vi "G2CPU Circle Lines.vi"(6 "Auto Release (Enabled)":T2={"Auto Release Amount of Lines (Enabled)"=TRUE, "Auto Release Center X (Enabled)"=TRUE, "Auto Release Center Y (Enabled)"=TRUE, "Auto Release Inner Radius (Enabled)"=TRUE, "Auto Release Outer Radius (Enabled)"=TRUE}, 8 "error in (no error)":errorcluster, 11 "Circles Parameters":T1) -> (0 "error out":errorcluster, 3 "Lines":T3)   [LabVIEW 2020, in "G2CPU Line Profile.lvlib"]
doc: "Create a set of points representing a set of Circles for image processing.\n\nPoints 1 on the output define the starting point of the lines and Points 2 define the stopping point of the lines.\nThe keys put out define the grouping of the lines to each circle."
uses:
  G2CPU Line Profile.lvlib
  <vilib>/Natan Biesmans/G2CPU GPU and CPU HPC Toolkit/G2CPU Libraries/Arrays/1DArray/f32/1D Array f32.lvclass
  C:/Program Files/National Instruments/LabVIEW 2025/vi.lib/Natan Biesmans/G2CPU GPU and CPU HPC Toolkit/G2CPU Libraries/Arrays/Array/Array Prototype.lvclass
  <vilib>/Natan Biesmans/G2CPU GPU and CPU HPC Toolkit/G2CPU Libraries/Arrays/1DArray/u32/1D Array u32.lvclass
  <vilib>/Natan Biesmans/G2CPU GPU and CPU HPC Toolkit/G2CPU Libraries/Arrays/1DArray/s32/1D Array s32.lvclass
  <vilib>/Natan Biesmans/G2CPU GPU and CPU HPC Toolkit/G2CPU Libraries/Arrays/Array/Array Prototype.lvclass/Array Prototype.ctl
  5b6760fa-9266-4741-afe7-4312c65416e9.vi
  3ad29c53-26f3-45f8-97d6-314157a676f7.vi
  14fba4ab-b554-44ef-a6f4-b6fd1a5d0cda.vi
  d3b3dbab-8883-4f98-9cce-319203c44813.vi
  e6c5d5d9-651a-47bf-ad11-961ed0f765a8.vi
  89c6f82f-ffef-4584-9d82-73d0fa6da3da.vi
  6a456209-1d8e-4cf0-9b04-3ffbd32bc9ac.vi
  96931e95-d0f5-44f7-b248-8357b3156dd5.vi
  d7ba55f0-9849-4505-a6fd-be5dcb5421fd.vi
  1cc5007f-c24b-4d5b-aa75-be27a96b3985.vi
  9a111955-ab15-448a-9318-e20ab5826a62.vi
  6db02158-8bc6-4d9a-a007-839d85d2f15d.vi
  ec8ba2e3-79c6-4f50-951d-f45e21c11e8a.vi
  f4669a4f-8dee-47e0-9080-20b8edd3c1cc.vi
  7ced169a-8142-4f3b-944f-65e1b7c596f5.vi
  2317dfd0-6b1c-49a0-9577-73dec4764c65.vi
  <vilib>/Natan Biesmans/G2CPU GPU and CPU HPC Toolkit/G2CPU Libraries/Arrays/Array/G2CPU Get Array Pointer.vi
  5b6760fa-9266-4741-afe7-4312c65416e9.vi/10d88d95-1d79-457d-a71e-58ed0fd5ba1c.vi
  3ad29c53-26f3-45f8-97d6-314157a676f7.vi/266dcd25-0bcc-42fd-b83c-a48544f38d1c.vi
  14fba4ab-b554-44ef-a6f4-b6fd1a5d0cda.vi/6197f869-f6d4-49b3-9b2c-cc979b422c2e.vi
  14fba4ab-b554-44ef-a6f4-b6fd1a5d0cda.vi/a7e86dbb-b4c0-485c-89c5-522e60ee265c.vi
  d3b3dbab-8883-4f98-9cce-319203c44813.vi/6197f869-f6d4-49b3-9b2c-cc979b422c2e.vi
  d3b3dbab-8883-4f98-9cce-319203c44813.vi/a7e86dbb-b4c0-485c-89c5-522e60ee265c.vi
  e6c5d5d9-651a-47bf-ad11-961ed0f765a8.vi/6197f869-f6d4-49b3-9b2c-cc979b422c2e.vi
  e6c5d5d9-651a-47bf-ad11-961ed0f765a8.vi/a7e86dbb-b4c0-485c-89c5-522e60ee265c.vi
  89c6f82f-ffef-4584-9d82-73d0fa6da3da.vi/6197f869-f6d4-49b3-9b2c-cc979b422c2e.vi
  89c6f82f-ffef-4584-9d82-73d0fa6da3da.vi/a7e86dbb-b4c0-485c-89c5-522e60ee265c.vi
  6a456209-1d8e-4cf0-9b04-3ffbd32bc9ac.vi/5793b77b-c002-4ebf-9075-685617c95341.vi
  6a456209-1d8e-4cf0-9b04-3ffbd32bc9ac.vi/2ed3ef86-c00d-4d71-b84c-20267a6dfcf9.vi
  96931e95-d0f5-44f7-b248-8357b3156dd5.vi/5793b77b-c002-4ebf-9075-685617c95341.vi
  96931e95-d0f5-44f7-b248-8357b3156dd5.vi/2ed3ef86-c00d-4d71-b84c-20267a6dfcf9.vi
  d7ba55f0-9849-4505-a6fd-be5dcb5421fd.vi/5793b77b-c002-4ebf-9075-685617c95341.vi
  d7ba55f0-9849-4505-a6fd-be5dcb5421fd.vi/2ed3ef86-c00d-4d71-b84c-20267a6dfcf9.vi
  1cc5007f-c24b-4d5b-aa75-be27a96b3985.vi/5793b77b-c002-4ebf-9075-685617c95341.vi
  1cc5007f-c24b-4d5b-aa75-be27a96b3985.vi/2ed3ef86-c00d-4d71-b84c-20267a6dfcf9.vi
  9a111955-ab15-448a-9318-e20ab5826a62.vi/e9bebd79-1c27-4fc1-b91f-30516104c7f0.vi
  6db02158-8bc6-4d9a-a007-839d85d2f15d.vi/7467a0f1-0650-4e63-b635-b3d2b2ec9a4e.vi
  6db02158-8bc6-4d9a-a007-839d85d2f15d.vi/8ee11bc3-5ef5-497e-97f0-8db2b3aaa149.vi
  6db02158-8bc6-4d9a-a007-839d85d2f15d.vi/c7af9698-5e3c-4e11-95da-3024075b67d2.vi
  ec8ba2e3-79c6-4f50-951d-f45e21c11e8a.vi/a7ec311c-7cd8-4650-9526-d70ff0a769d1.vi
  f4669a4f-8dee-47e0-9080-20b8edd3c1cc.vi/e9bebd79-1c27-4fc1-b91f-30516104c7f0.vi
  7ced169a-8142-4f3b-944f-65e1b7c596f5.vi/7467a0f1-0650-4e63-b635-b3d2b2ec9a4e.vi
  7ced169a-8142-4f3b-944f-65e1b7c596f5.vi/8ee11bc3-5ef5-497e-97f0-8db2b3aaa149.vi
  7ced169a-8142-4f3b-944f-65e1b7c596f5.vi/c7af9698-5e3c-4e11-95da-3024075b67d2.vi
  2317dfd0-6b1c-49a0-9577-73dec4764c65.vi/2e03f477-51b7-4ba0-bb4f-4f838f6557e6.vi
  2317dfd0-6b1c-49a0-9577-73dec4764c65.vi/125d45d4-836b-469d-8a4a-6adb452f866d.vi
  2317dfd0-6b1c-49a0-9577-73dec4764c65.vi/8038e9ed-2e71-4568-91ba-0d873494c5ed.vi
  14fba4ab-b554-44ef-a6f4-b6fd1a5d0cda.vi/6197f869-f6d4-49b3-9b2c-cc979b422c2e.vi/3e802c67-fb96-46a3-ae13-4994a8508b4f.vi
  14fba4ab-b554-44ef-a6f4-b6fd1a5d0cda.vi/6197f869-f6d4-49b3-9b2c-cc979b422c2e.vi/5a50fc67-79e7-4972-80c2-92243cd53dd4.vi
  14fba4ab-b554-44ef-a6f4-b6fd1a5d0cda.vi/a7e86dbb-b4c0-485c-89c5-522e60ee265c.vi/730f6c57-5c0b-4ee9-b61e-75067b25222b.vi
  14fba4ab-b554-44ef-a6f4-b6fd1a5d0cda.vi/a7e86dbb-b4c0-485c-89c5-522e60ee265c.vi/096b8799-7810-404e-baca-ba9279cec4bd.vi
  14fba4ab-b554-44ef-a6f4-b6fd1a5d0cda.vi/a7e86dbb-b4c0-485c-89c5-522e60ee265c.vi/0f1a5a47-bcc5-4796-ac31-8dfcfbc0d7d1.vi
  14fba4ab-b554-44ef-a6f4-b6fd1a5d0cda.vi/a7e86dbb-b4c0-485c-89c5-522e60ee265c.vi/89f12e17-3330-4b72-ad8f-8dd636660732.vi
  d3b3dbab-8883-4f98-9cce-319203c44813.vi/6197f869-f6d4-49b3-9b2c-cc979b422c2e.vi/3e802c67-fb96-46a3-ae13-4994a8508b4f.vi
  d3b3dbab-8883-4f98-9cce-319203c44813.vi/6197f869-f6d4-49b3-9b2c-cc979b422c2e.vi/5a50fc67-79e7-4972-80c2-92243cd53dd4.vi
  d3b3dbab-8883-4f98-9cce-319203c44813.vi/a7e86dbb-b4c0-485c-89c5-522e60ee265c.vi/730f6c57-5c0b-4ee9-b61e-75067b25222b.vi
  d3b3dbab-8883-4f98-9cce-319203c44813.vi/a7e86dbb-b4c0-485c-89c5-522e60ee265c.vi/096b8799-7810-404e-baca-ba9279cec4bd.vi
  d3b3dbab-8883-4f98-9cce-319203c44813.vi/a7e86dbb-b4c0-485c-89c5-522e60ee265c.vi/0f1a5a47-bcc5-4796-ac31-8dfcfbc0d7d1.vi
  d3b3dbab-8883-4f98-9cce-319203c44813.vi/a7e86dbb-b4c0-485c-89c5-522e60ee265c.vi/89f12e17-3330-4b72-ad8f-8dd636660732.vi
  e6c5d5d9-651a-47bf-ad11-961ed0f765a8.vi/6197f869-f6d4-49b3-9b2c-cc979b422c2e.vi/3e802c67-fb96-46a3-ae13-4994a8508b4f.vi
  e6c5d5d9-651a-47bf-ad11-961ed0f765a8.vi/6197f869-f6d4-49b3-9b2c-cc979b422c2e.vi/5a50fc67-79e7-4972-80c2-92243cd53dd4.vi
  e6c5d5d9-651a-47bf-ad11-961ed0f765a8.vi/a7e86dbb-b4c0-485c-89c5-522e60ee265c.vi/730f6c57-5c0b-4ee9-b61e-75067b25222b.vi
  e6c5d5d9-651a-47bf-ad11-961ed0f765a8.vi/a7e86dbb-b4c0-485c-89c5-522e60ee265c.vi/096b8799-7810-404e-baca-ba9279cec4bd.vi
  e6c5d5d9-651a-47bf-ad11-961ed0f765a8.vi/a7e86dbb-b4c0-485c-89c5-522e60ee265c.vi/0f1a5a47-bcc5-4796-ac31-8dfcfbc0d7d1.vi
  e6c5d5d9-651a-47bf-ad11-961ed0f765a8.vi/a7e86dbb-b4c0-485c-89c5-522e60ee265c.vi/89f12e17-3330-4b72-ad8f-8dd636660732.vi
  89c6f82f-ffef-4584-9d82-73d0fa6da3da.vi/6197f869-f6d4-49b3-9b2c-cc979b422c2e.vi/3e802c67-fb96-46a3-ae13-4994a8508b4f.vi
  89c6f82f-ffef-4584-9d82-73d0fa6da3da.vi/6197f869-f6d4-49b3-9b2c-cc979b422c2e.vi/5a50fc67-79e7-4972-80c2-92243cd53dd4.vi
  89c6f82f-ffef-4584-9d82-73d0fa6da3da.vi/a7e86dbb-b4c0-485c-89c5-522e60ee265c.vi/730f6c57-5c0b-4ee9-b61e-75067b25222b.vi
  89c6f82f-ffef-4584-9d82-73d0fa6da3da.vi/a7e86dbb-b4c0-485c-89c5-522e60ee265c.vi/096b8799-7810-404e-baca-ba9279cec4bd.vi
  89c6f82f-ffef-4584-9d82-73d0fa6da3da.vi/a7e86dbb-b4c0-485c-89c5-522e60ee265c.vi/0f1a5a47-bcc5-4796-ac31-8dfcfbc0d7d1.vi
  89c6f82f-ffef-4584-9d82-73d0fa6da3da.vi/a7e86dbb-b4c0-485c-89c5-522e60ee265c.vi/89f12e17-3330-4b72-ad8f-8dd636660732.vi
  6a456209-1d8e-4cf0-9b04-3ffbd32bc9ac.vi/5793b77b-c002-4ebf-9075-685617c95341.vi/3e802c67-fb96-46a3-ae13-4994a8508b4f.vi
  6a456209-1d8e-4cf0-9b04-3ffbd32bc9ac.vi/5793b77b-c002-4ebf-9075-685617c95341.vi/5a50fc67-79e7-4972-80c2-92243cd53dd4.vi
  6a456209-1d8e-4cf0-9b04-3ffbd32bc9ac.vi/2ed3ef86-c00d-4d71-b84c-20267a6dfcf9.vi/730f6c57-5c0b-4ee9-b61e-75067b25222b.vi
  6a456209-1d8e-4cf0-9b04-3ffbd32bc9ac.vi/2ed3ef86-c00d-4d71-b84c-20267a6dfcf9.vi/096b8799-7810-404e-baca-ba9279cec4bd.vi
  6a456209-1d8e-4cf0-9b04-3ffbd32bc9ac.vi/2ed3ef86-c00d-4d71-b84c-20267a6dfcf9.vi/0f1a5a47-bcc5-4796-ac31-8dfcfbc0d7d1.vi
  6a456209-1d8e-4cf0-9b04-3ffbd32bc9ac.vi/2ed3ef86-c00d-4d71-b84c-20267a6dfcf9.vi/89f12e17-3330-4b72-ad8f-8dd636660732.vi
  96931e95-d0f5-44f7-b248-8357b3156dd5.vi/5793b77b-c002-4ebf-9075-685617c95341.vi/3e802c67-fb96-46a3-ae13-4994a8508b4f.vi
  96931e95-d0f5-44f7-b248-8357b3156dd5.vi/5793b77b-c002-4ebf-9075-685617c95341.vi/5a50fc67-79e7-4972-80c2-92243cd53dd4.vi
  96931e95-d0f5-44f7-b248-8357b3156dd5.vi/2ed3ef86-c00d-4d71-b84c-20267a6dfcf9.vi/730f6c57-5c0b-4ee9-b61e-75067b25222b.vi
  96931e95-d0f5-44f7-b248-8357b3156dd5.vi/2ed3ef86-c00d-4d71-b84c-20267a6dfcf9.vi/096b8799-7810-404e-baca-ba9279cec4bd.vi
  96931e95-d0f5-44f7-b248-8357b3156dd5.vi/2ed3ef86-c00d-4d71-b84c-20267a6dfcf9.vi/0f1a5a47-bcc5-4796-ac31-8dfcfbc0d7d1.vi
  96931e95-d0f5-44f7-b248-8357b3156dd5.vi/2ed3ef86-c00d-4d71-b84c-20267a6dfcf9.vi/89f12e17-3330-4b72-ad8f-8dd636660732.vi
  d7ba55f0-9849-4505-a6fd-be5dcb5421fd.vi/5793b77b-c002-4ebf-9075-685617c95341.vi/3e802c67-fb96-46a3-ae13-4994a8508b4f.vi
  d7ba55f0-9849-4505-a6fd-be5dcb5421fd.vi/5793b77b-c002-4ebf-9075-685617c95341.vi/5a50fc67-79e7-4972-80c2-92243cd53dd4.vi
  d7ba55f0-9849-4505-a6fd-be5dcb5421fd.vi/2ed3ef86-c00d-4d71-b84c-20267a6dfcf9.vi/730f6c57-5c0b-4ee9-b61e-75067b25222b.vi
  d7ba55f0-9849-4505-a6fd-be5dcb5421fd.vi/2ed3ef86-c00d-4d71-b84c-20267a6dfcf9.vi/096b8799-7810-404e-baca-ba9279cec4bd.vi
  d7ba55f0-9849-4505-a6fd-be5dcb5421fd.vi/2ed3ef86-c00d-4d71-b84c-20267a6dfcf9.vi/0f1a5a47-bcc5-4796-ac31-8dfcfbc0d7d1.vi
  d7ba55f0-9849-4505-a6fd-be5dcb5421fd.vi/2ed3ef86-c00d-4d71-b84c-20267a6dfcf9.vi/89f12e17-3330-4b72-ad8f-8dd636660732.vi
  1cc5007f-c24b-4d5b-aa75-be27a96b3985.vi/5793b77b-c002-4ebf-9075-685617c95341.vi/3e802c67-fb96-46a3-ae13-4994a8508b4f.vi
  1cc5007f-c24b-4d5b-aa75-be27a96b3985.vi/5793b77b-c002-4ebf-9075-685617c95341.vi/5a50fc67-79e7-4972-80c2-92243cd53dd4.vi
  1cc5007f-c24b-4d5b-aa75-be27a96b3985.vi/2ed3ef86-c00d-4d71-b84c-20267a6dfcf9.vi/730f6c57-5c0b-4ee9-b61e-75067b25222b.vi
  1cc5007f-c24b-4d5b-aa75-be27a96b3985.vi/2ed3ef86-c00d-4d71-b84c-20267a6dfcf9.vi/096b8799-7810-404e-baca-ba9279cec4bd.vi
  1cc5007f-c24b-4d5b-aa75-be27a96b3985.vi/2ed3ef86-c00d-4d71-b84c-20267a6dfcf9.vi/0f1a5a47-bcc5-4796-ac31-8dfcfbc0d7d1.vi
  1cc5007f-c24b-4d5b-aa75-be27a96b3985.vi/2ed3ef86-c00d-4d71-b84c-20267a6dfcf9.vi/89f12e17-3330-4b72-ad8f-8dd636660732.vi
  2317dfd0-6b1c-49a0-9577-73dec4764c65.vi/2e03f477-51b7-4ba0-bb4f-4f838f6557e6.vi/d8e2d9cc-c923-495e-b121-b6b84788c73f.vi
  2317dfd0-6b1c-49a0-9577-73dec4764c65.vi/2e03f477-51b7-4ba0-bb4f-4f838f6557e6.vi/345e91f0-9a5e-4de4-af9c-133346717e4a.vi
  <vilib>/Natan Biesmans/G2CPU GPU and CPU HPC Toolkit/G2CPU Libraries/Arrays/2DArray/f32/2D Array f32.lvclass
  <vilib>/Natan Biesmans/G2CPU GPU and CPU HPC Toolkit/G2CPU Libraries/Arrays/2DArray/binary/2D Array binary.lvclass
  <vilib>/Natan Biesmans/G2CPU GPU and CPU HPC Toolkit/G2CPU Libraries/Arrays/1DArray/binary/1D Array binary.lvclass
  <vilib>/Natan Biesmans/G2CPU GPU and CPU HPC Toolkit/G2CPU Libraries/Arrays/2DArray/u32/2D Array u32.lvclass
  <vilib>/Natan Biesmans/G2CPU GPU and CPU HPC Toolkit/ArrayFire Driver/VIs/cos.vi
  <vilib>/Natan Biesmans/G2CPU GPU and CPU HPC Toolkit/G2CPU Libraries/Arrays/Array/G2CPU Set Array Pointer.vi
  <vilib>/Natan Biesmans/G2CPU GPU and CPU HPC Toolkit/ArrayFire Driver/VIs/sin.vi
  <vilib>/Natan Biesmans/G2CPU GPU and CPU HPC Toolkit/G2CPU Libraries/Arrays/SubVI/is 2D.vi
  <vilib>/Natan Biesmans/G2CPU GPU and CPU HPC Toolkit/ArrayFire Driver/VIs/mul.vi
  <vilib>/Natan Biesmans/G2CPU GPU and CPU HPC Toolkit/ArrayFire Driver/VIs/add.vi
  <vilib>/Natan Biesmans/G2CPU GPU and CPU HPC Toolkit/ArrayFire Driver/VIs/transpose.vi
  <vilib>/Natan Biesmans/G2CPU GPU and CPU HPC Toolkit/ArrayFire Driver/VIs/flat.vi
  <vilib>/Natan Biesmans/G2CPU GPU and CPU HPC Toolkit/ArrayFire Driver/VIs/where.vi
  <vilib>/Natan Biesmans/G2CPU GPU and CPU HPC Toolkit/ArrayFire Driver/VIs/cast.vi
  <vilib>/Natan Biesmans/G2CPU GPU and CPU HPC Toolkit/ArrayFire Driver/VIs/lookup.vi
  <vilib>/Natan Biesmans/G2CPU GPU and CPU HPC Toolkit/G2CPU Libraries/Arrays/Array/Array Prototype.lvclass
  <vilib>/Natan Biesmans/G2CPU GPU and CPU HPC Toolkit/G2CPU Libraries/Arrays/DataTypes/f32/f32.lvclass
  <vilib>/Natan Biesmans/G2CPU GPU and CPU HPC Toolkit/G2CPU Libraries/Arrays/2DArray/2D Array Prototype.lvclass
  <vilib>/Natan Biesmans/G2CPU GPU and CPU HPC Toolkit/G2CPU Libraries/Arrays/1DArray/1D Array Prototype.lvclass
  <vilib>/Natan Biesmans/G2CPU GPU and CPU HPC Toolkit/G2CPU Libraries/Arrays/DataTypes/Boolean/Boolean.lvclass
  <vilib>/Natan Biesmans/G2CPU GPU and CPU HPC Toolkit/G2CPU Libraries/Arrays/DataTypes/U32/U32.lvclass
  <vilib>/Natan Biesmans/G2CPU GPU and CPU HPC Toolkit/G2CPU Libraries/Arrays/DataTypes/I32/s32.lvclass
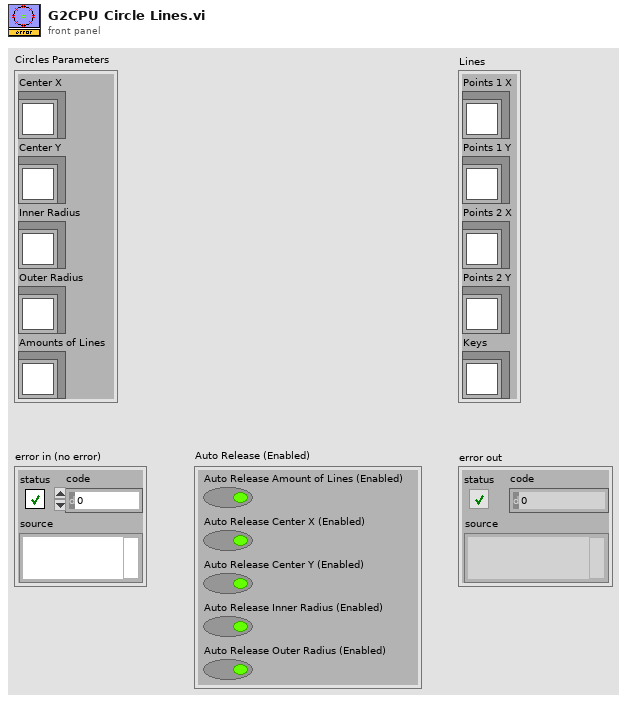
[diagram p1: front panel]
types:
  T1 = cluster{"Center X":refnum<class "1D Array f32.lvclass">, "Center Y":refnum<class "1D Array f32.lvclass">, "Inner Radius":refnum<class "1D Array f32.lvclass">, "Outer Radius":refnum<class "1D Array f32.lvclass">, "Amounts of Lines":refnum<class "1D Array s32.lvclass">}
  T2 = cluster{"Auto Release Amount of Lines (Enabled)":bool, "Auto Release Center X (Enabled)":bool, "Auto Release Center Y (Enabled)":bool, "Auto Release Inner Radius (Enabled)":bool, "Auto Release Outer Radius (Enabled)":bool}
  T3 = cluster{"Points 1 X":refnum<class "1D Array f32.lvclass">, "Points 1 Y":refnum<class "1D Array f32.lvclass">, "Points 2 X":refnum<class "1D Array f32.lvclass">, "Points 2 Y":refnum<class "1D Array f32.lvclass">, "Keys":refnum<class "1D Array u32.lvclass">}
  T4 = cluster{"Px 1":refnum<class "1D Array f32.lvclass">, "Py 1":refnum<class "1D Array f32.lvclass">, "Px 2":refnum<class "1D Array f32.lvclass">, "Py 2":refnum<class "1D Array f32.lvclass">, "Keys":refnum<class "1D Array u32.lvclass">}
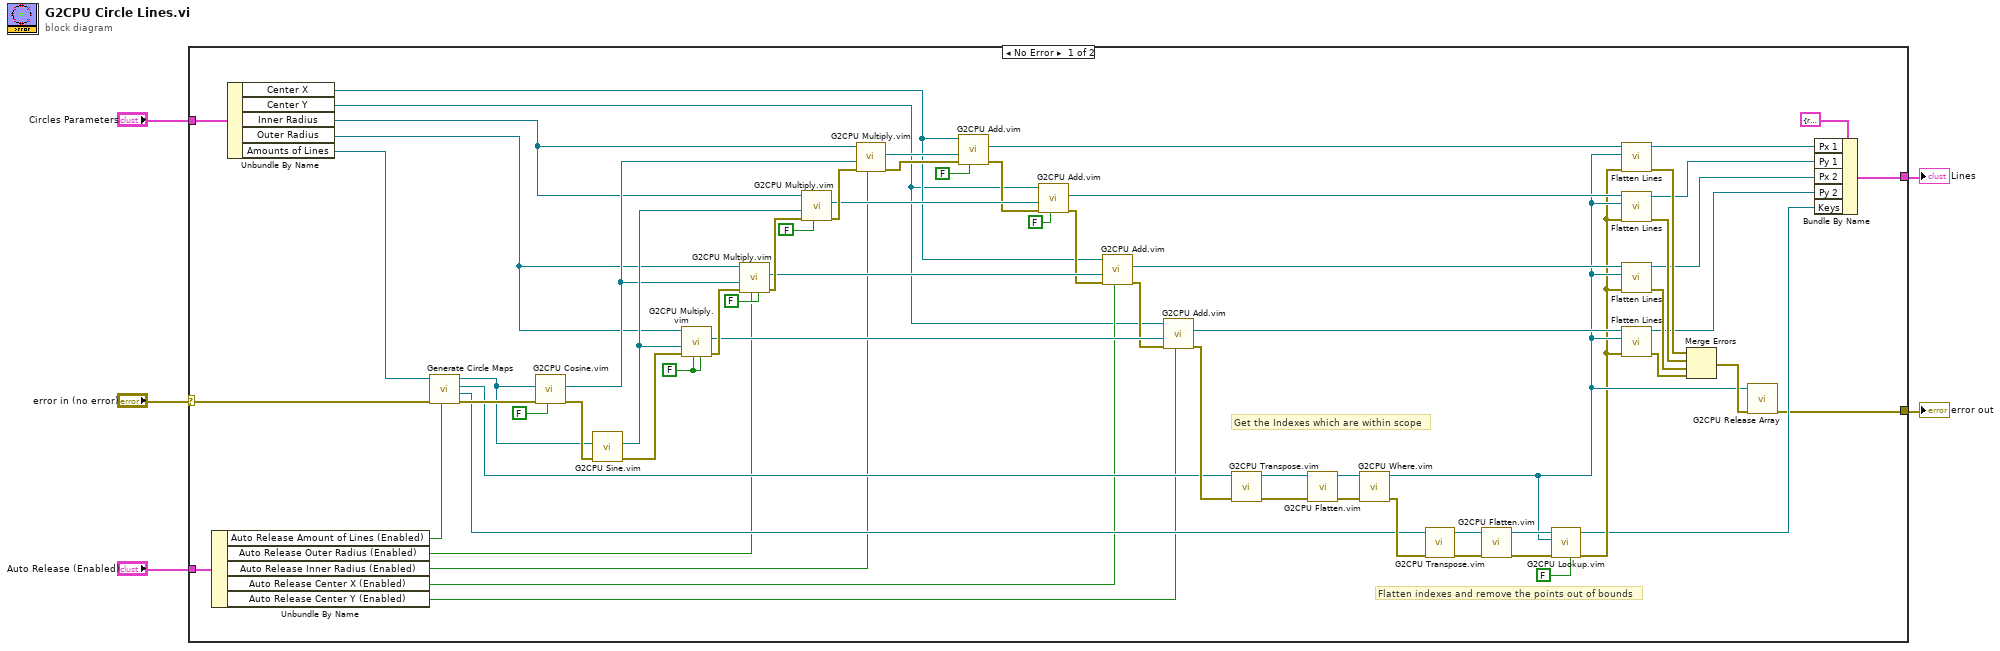
[diagram p0: block diagram]
diagram:
  n1 = case shown="No Error" "error in (no error)" {
    selector: "error in (no error)" -> [w20 _]
    tunnel: [w19 _] -> w4
    tunnel: [w18 _] -> w3
    tunnel: "Auto Release (Enabled)" -> [w17 _]
    tunnel: "Circles Parameters" -> [w11 _]
    frame No Error {
      w65 = FALSE ("Auto Release lhs")
      # "Flatten indexes and remove the points out of bounds"
      # "Get the Indexes which are within scope"
      n2 = Unbundle By Name(w17) -> ("Auto Release Amount of Lines (Enabled)"=w16:bool, "Auto Release Outer Radius (Enabled)"=w14:bool, "Auto Release Inner Radius (Enabled)"=w15:bool, "Auto Release Center X (Enabled)"=w13:bool, "Auto Release Center Y (Enabled)"=w12:bool)
      n3 = Unbundle By Name(w11) -> ("Center X"=w10:refnum<class "1D Array f32.lvclass">, "Center Y"=w9:refnum<class "1D Array f32.lvclass">, "Inner Radius"=w8:refnum<class "1D Array f32.lvclass">, "Outer Radius"=w7:refnum<class "1D Array f32.lvclass">, "Amounts of Lines"=w6:refnum<class "1D Array s32.lvclass">)
      n4 = call "Generate Circle Maps.vi"("Auto Release Amount of Lines (Enabled)"=w16, "error in (no error)"=w20, "Amount of Lines"=w6) -> ("error out"=w73:errorcluster, "Keys"=w21:refnum<class "2D Array u32.lvclass">, "Point mask within bounds"=w22:refnum<class "2D Array binary.lvclass">, "Circle Scales"=w23:refnum<class "2D Array f32.lvclass">)  [unwired: 5 in]
      n5 = call "G2CPU Cosine.vim"("Auto Release (Enabled)"=FALSE, "error in (no error)"=w73, "Array in"=w23) -> ("error out"=w72:errorcluster, "Array Result"=w69:refnum<class "2D Array f32.lvclass">)  [unwired: 7 in]
      n6 = call "G2CPU Sine.vim"("error in (no error)"=w72, "Array in"=w23) -> ("error out"=w68:errorcluster, "Array Result"=w70:refnum<class "2D Array f32.lvclass">)  [unwired: 8 in]
      n7 = call "G2CPU Multiply.vim"("Auto Release rhs"=w65, "Auto Release lhs"=w65, "error in (no error)"=w68, "Array rhs"=w70, "Array lhs"=w7) -> ("error out"=w67:errorcluster, "Array Result"=w58:refnum<class "2D Array f32.lvclass">)  [unwired: 5 in]
      n8 = call "G2CPU Multiply.vim"("Auto Release rhs"=FALSE, "Auto Release lhs"=w14, "error in (no error)"=w67, "Array rhs"=w69, "Array lhs"=w7) -> ("error out"=w66:errorcluster, "Array Result"=w59:refnum<class "2D Array f32.lvclass">)  [unwired: 5 in]
      n9 = call "G2CPU Multiply.vim"("Auto Release lhs"=FALSE, "error in (no error)"=w66, "Array rhs"=w70, "Array lhs"=w8) -> ("error out"=w62:errorcluster, "Array Result"=w60:refnum<class "2D Array f32.lvclass">)  [unwired: 6 in]
      n10 = call "G2CPU Multiply.vim"("Auto Release lhs"=w15, "error in (no error)"=w62, "Array rhs"=w69, "Array lhs"=w8) -> ("error out"=w57:errorcluster, "Array Result"=w61:refnum<class "2D Array f32.lvclass">)  [unwired: 6 in]
      n11 = call "G2CPU Add.vim"("Auto Release lhs (Enabled)"=FALSE, "error in (no error)"=w57, "Array rhs"=w61, "Array lhs"=w10) -> ("error out"=w56:errorcluster, "Array Result"=w48:refnum<class "2D Array f32.lvclass">)  [unwired: 6 in]
      n12 = call "G2CPU Add.vim"("Auto Release lhs (Enabled)"=FALSE, "error in (no error)"=w56, "Array rhs"=w60, "Array lhs"=w9) -> ("error out"=w55:errorcluster, "Array Result"=w49:refnum<class "2D Array f32.lvclass">)  [unwired: 6 in]
      n13 = call "G2CPU Add.vim"("Auto Release lhs (Enabled)"=w13, "error in (no error)"=w55, "Array rhs"=w59, "Array lhs"=w10) -> ("error out"=w54:errorcluster, "Array Result"=w50:refnum<class "2D Array f32.lvclass">)  [unwired: 6 in]
      n14 = call "G2CPU Add.vim"("Auto Release lhs (Enabled)"=w12, "error in (no error)"=w54, "Array rhs"=w58, "Array lhs"=w9) -> ("error out"=w30:errorcluster, "Array Result"=w51:refnum<class "2D Array f32.lvclass">)  [unwired: 6 in]
      n15 = call "G2CPU Transpose.vim"("error in (no error)"=w30, "Array In"=w22) -> ("error out"=w36:errorcluster, "Array out"=w46:refnum<class "2D Array binary.lvclass">)  [unwired: 8 in]
      n16 = call "G2CPU Flatten.vim"("error in (no error)"=w36, "Array In"=w46) -> ("error out"=w35:errorcluster, "Array out"=w45:refnum<class "1D Array binary.lvclass">)  [unwired: 8 in]
      n17 = call "G2CPU Where.vim"("error in (no error)"=w35, "Array in"=w45) -> ("error out"=w32:errorcluster, "Non Zero Indices"=w37:refnum<class "1D Array u32.lvclass">)  [unwired: 8 in]
      n18 = call "G2CPU Transpose.vim"("error in (no error)"=w32, "Array In"=w21) -> ("error out"=w34:errorcluster, "Array out"=w47:refnum<class "2D Array u32.lvclass">)  [unwired: 8 in]
      n19 = call "G2CPU Flatten.vim"("error in (no error)"=w34, "Array In"=w47) -> ("error out"=w33:errorcluster, "Array out"=w43:refnum<class "1D Array u32.lvclass">)  [unwired: 8 in]
      n20 = call "G2CPU Lookup.vim"("Auto Release Indices (Enabled)"=FALSE, "error in (no error)"=w33, "Indices (1D)"=w37, "Array In"=w43) -> ("error out"=w31:errorcluster, "Indexed Array"=w24:refnum<class "1D Array u32.lvclass">)  [unwired: 6 in]
      n21 = call "Flatten Lines.vi"("error in (no error)"=w31, "Valid Point Indexes (flattened)"=w37, "Lines In"=w48) -> ("error out"=w42:errorcluster, "Flattened Lines Out"=w28:refnum<class "1D Array f32.lvclass">)  [unwired: 7 in]
      n22 = call "Flatten Lines.vi"("error in (no error)"=w31, "Valid Point Indexes (flattened)"=w37, "Lines In"=w49) -> ("error out"=w41:errorcluster, "Flattened Lines Out"=w27:refnum<class "1D Array f32.lvclass">)  [unwired: 7 in]
      n23 = call "Flatten Lines.vi"("error in (no error)"=w31, "Valid Point Indexes (flattened)"=w37, "Lines In"=w50) -> ("error out"=w40:errorcluster, "Flattened Lines Out"=w26:refnum<class "1D Array f32.lvclass">)  [unwired: 7 in]
      n24 = call "Flatten Lines.vi"("error in (no error)"=w31, "Valid Point Indexes (flattened)"=w37, "Lines In"=w51) -> ("error out"=w39:errorcluster, "Flattened Lines Out"=w25:refnum<class "1D Array f32.lvclass">)  [unwired: 7 in]
      n25 = Merge Errors(w42, w41, w40, w39) -> (w38:errorcluster)
      n26 = call <vilib>:"G2CPU Release Array.vi"("error in (no error)"=w38, "Array in"=w37) -> ("error out"=w19:errorcluster)  [unwired: 9 in]
      n27 = Bundle By Name(cluster=T4 {"Px 1"=refnum, "Py 1"=refnum, "Px 2"=refnum, "Py 2"=refnum, "Keys"=refnum} ("Cluster"), "Px 1"=w28, "Py 1"=w27, "Px 2"=w26, "Py 2"=w25, "Keys"=w24) -> (w18:T4)
    }
    frame Error {
    }
  }
  "error out" <- w4
  "Lines" <- w3
